vi "Main Engine Stream Process.vi"(8 "error in (no error)":errorcluster, 10 "Refs":T1 {"Port Settings"."FD ISO Mode" items=["ISO", "Non ISO", "ISO Legacy"]; "Port Settings"."Termination" items=["Off", "On"]; "Port Settings"."Mode" items=["CAN 2.0", "CAN FD", "CAN FD+BRS"]}, 11 "Process in":refnum<class "Process.lvclass">=refnum) -> (0 "error out":errorcluster)   [LabVIEW 2021, in "CAN Stream Support Engine.lvlib"]
uses:
  CAN Stream Support Engine.lvlib
  Types/Engine Stream State.ctl
  <vilib>/xnet/xnet.llb/XNET Frame Type CAN.ctl
  <vilib>/xnet/xnet.llb/XNET Frame CAN.ctl
  <resource>/objmgr/xnet.rc
  <vilib>/xnet/xnet.llb/XNET CAN Last Err.ctl
  <vilib>/xnet/xnet.llb/XNET CAN Comm State.ctl
  <vilib>/xnet/xnet.llb/XNET CAN Comm.ctl
  Addon Shared/Types/Stream Type.ctl
  Addon Shared/CAN Stream Support Shared.lvlib
  <vilib>/xnet/xnet.llb/XNET Create Session (Frame Input Stream).vi
  <vilib>/xnet/xnet.llb/XNET Read (State CAN Comm).vi
  <vilib>/xnet/xnet.llb/XNET Read (Frame CAN).vi
  <vilib>/NI/NIVS Inline Async API/_VS Inline Async API/Process/Process.lvclass
  Types/Engine Stream Refs.ctl
  Addon Shared/Types/Type Filter.ctl
  Addon Shared/Types/Direction Filter.ctl
  Addon Shared/Types/Filter Parameters.ctl
  Types/Engine Stream Port Settings.ctl
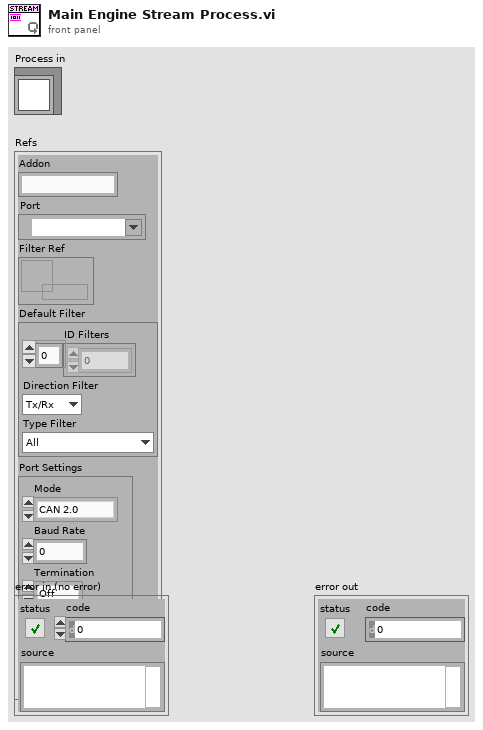
[diagram p1: front panel]
types:
  T1 = typedef "CAN Stream Support Engine.lvlib/Engine Stream Refs.ctl" = cluster{"Addon":string, "Port":refnum<k21>, "Filter Ref":refnum<data-value>, "Default Filter":T2, "Port Settings":T5}
  T2 = typedef "CAN Stream Support Shared.lvlib/Filter Parameters.ctl" = cluster{"ID Filters":u32[], "Direction Filter":T3, "Type Filter":T4}
  T3 = typedef "CAN Stream Support Shared.lvlib/Direction Filter.ctl" = enum16{"Tx/Rx", "Rx", "Tx"}
  T4 = typedef "CAN Stream Support Shared.lvlib/Type Filter.ctl" = enum16{"All", "CAN Data", "CAN Remote", "CAN Bus Error", "CAN 2.0 Data", "CAN FD Data", "CAN FD+BRS Data", "J1939 Data", "Delay", "Log Trigger", "Start Trigger"}
  T5 = typedef "CAN Stream Support Engine.lvlib/Engine Stream Port Settings.ctl" = cluster{"Mode":u32, "Baud Rate":u64, "Termination":u32, "FD ISO Mode":u32, "FD Baud Rate":u64}
  T6 = typedef "CAN Stream Support Engine.lvlib/Engine Stream State.ctl" = enum8{"Check for Connection", "Open XNET Session", "Publish", "Cleanup", "Exit"}
  T7 = typedef "CAN Stream Support Shared.lvlib/Stream Type.ctl" = cluster{"State":T8, "Frames":T11[]}
  T8 = typedef "XNET CAN Comm.ctl" = cluster{"fault code":i32, "fault?":bool, "communication state":T9, "last error":T10, "receive error counter":u8, "transmit error counter":u8, "transceiver error?":bool, "sleep?":bool}
  T9 = typedef "XNET CAN Comm State.ctl" = u8
  T10 = typedef "XNET CAN Last Err.ctl" = u8
  T11 = typedef "XNET Frame CAN.ctl" = cluster{"timestamp":timestamp, "payload":u8[], "identifier":u32, "type":T12, "extended?":bool, "echo?":bool}
  T12 = typedef "XNET Frame Type CAN.ctl" = u8
  T13 = cluster{"ID Filters":u32[], "Direction Filter":T3, "Type Filter":T4}
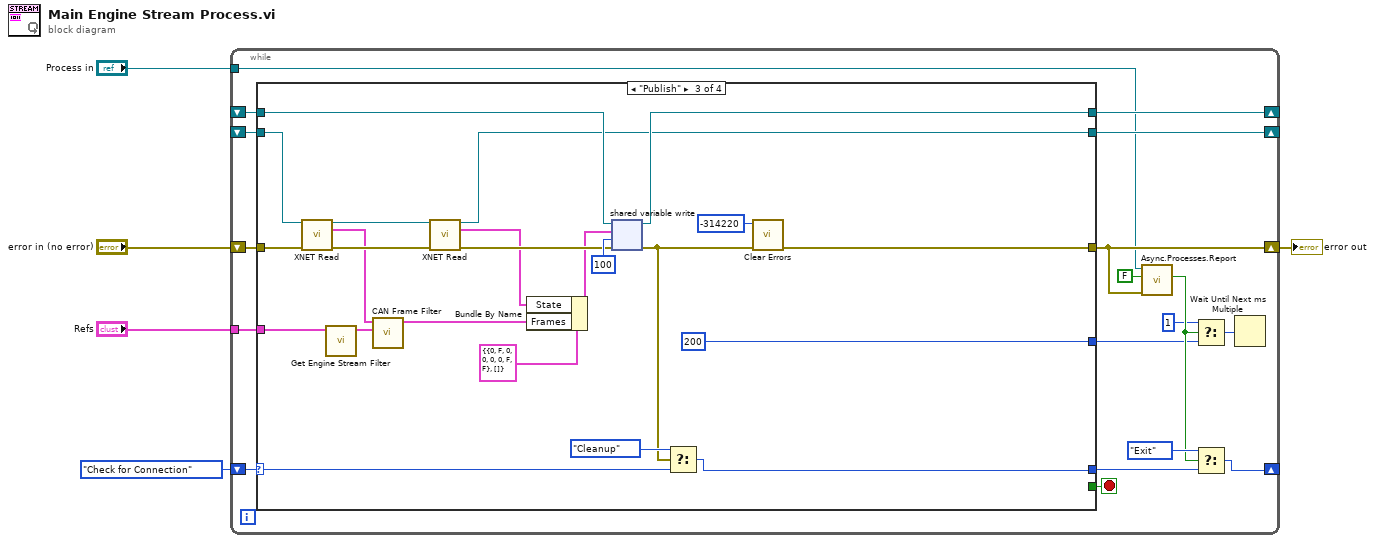
[diagram p0: block diagram]
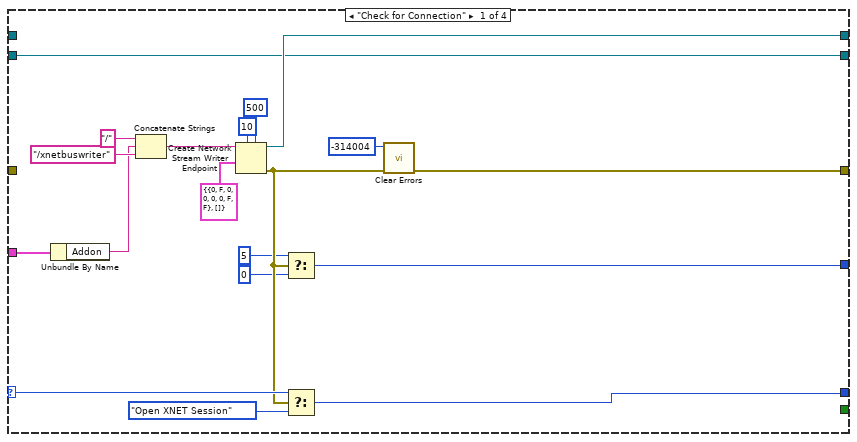
[diagram p2: hidden frame]
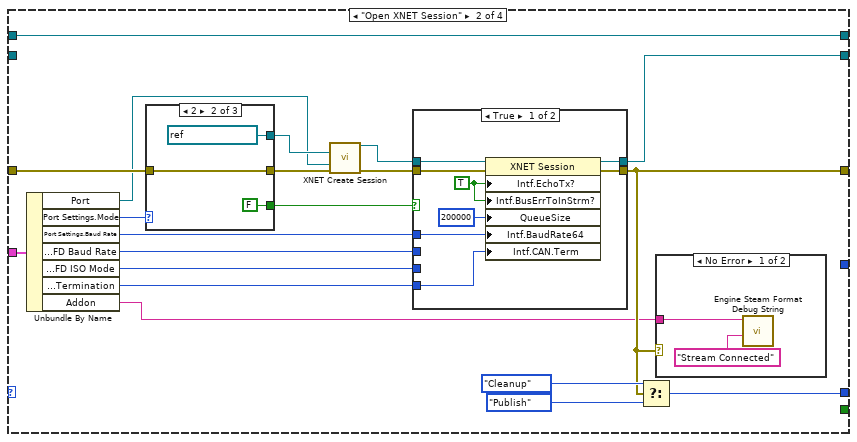
[diagram p3: hidden frame]
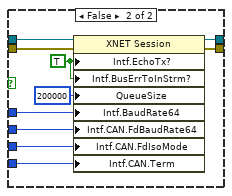
[diagram p4: hidden frame]
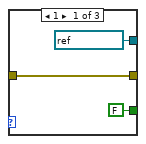
[diagram p5: hidden frame]
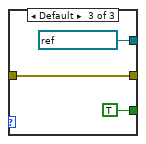
[diagram p6: hidden frame]
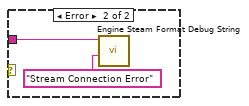
[diagram p7: hidden frame]
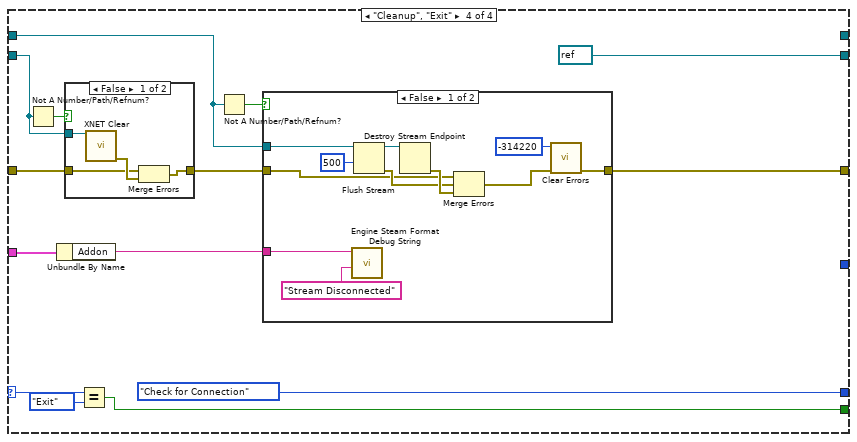
[diagram p8: hidden frame]
diagram:
  n1 = while {
    shift-right: [w11] -> _
    shift-left: Engine_Stream_State."Check for Connection" -> [w23]
    shift-right: [w22] -> _
    shift-left: _ -> [w21]
    shift-right: [w16] -> w3
    shift-left: "error in (no error)" -> [w20]
    shift-right: [w18] -> _
    shift-left: _ -> [w17]
    tunnel: "Process in" -> [w13]
    tunnel: "Refs" -> [w12]
    stop <- w19 stop-if-true
    n2 = case shown="\"Publish\"" w23 {
      selector: w23 -> [w40 _ w113 w129]
      tunnel: [w38 w59 w112 Engine_Stream_State."Check for Connection"] -> w14
      tunnel: [w37 w60 w114 _] -> w22
      tunnel: w21 -> [_ w60 w115 w126]
      tunnel: [w35 w55 w97 w119] -> w16
      tunnel: w20 -> [_ w46 w108 w121]
      tunnel: [_ _ _ w127] -> w19
      tunnel: [w36 w57 w103 refnum<k21> refnum ("session out")] -> w18
      tunnel: w17 -> [w36 _ w110 w123]
      tunnel: [w29 _ u32 200 ("millisecond multiple") _] -> w9
      tunnel: w12 -> [w25 w54 w107 w118]
      frame "Check for Connection" {
        n3 = Unbundle By Name(w25) -> ("Addon"=w24:string)
        n4 = Concatenate Strings("/" ("string"), w24, "/xnetbuswriter" ("reader url")) -> (w26:string)
        n5 = Create Network Stream Writer Endpoint(5:500 ("timeout in ms (-1)"), 7:10 ("writer buffer size"), 9:T7 {"State"={"fault code"=0, "fault?"=FALSE, "communication state"=0, "last error"=0, "receive error counter"=0, "transmit error counter"=0, "transceiver error?"=FALSE, "sleep?"=FALSE}, "Frames"=[]} ("Stream"), 11:w26) -> (0:w32:errorcluster, 3:w37:refnum<k21>)  [unwired: 3 in]
        n6 = Select(t=u32 5 ("millisecond multiple"), s=w32, f=u32 0) -> (s? t:f=w29:u32)
        n7 = Select(t=w40, s=w32, f=Engine_Stream_State."Open XNET Session") -> (s? t:f=w38:T6)
        n8 = call <vilib>:"Clear Errors.vi"("error in (no error)"=w32, "specific error code to clear (0: all)"=-314004) -> ("error out"=w35:errorcluster)  [unwired: 4 in, 1 out]
      }
      frame "Open XNET Session" {
        n9 = Unbundle By Name(w54) -> ("Port"=w43:refnum<k21>, "Port Settings.Mode"=w47:u32, "Port Settings.Baud Rate"=w45:u64, "Port Settings.FD Baud Rate"=w44:u64, "Port Settings.FD ISO Mode"=w48:u32, "Port Settings.Termination"=w52:u32, "Addon"=w53:string)
        n10 = case shown="2" w47 {
          tunnel: [refnum<k21> ":can_fd:" ("cluster (:memory:)") refnum<k21> ":can_fd_brs:" ("cluster (:memory:)") refnum<k21> ":memory:" ("cluster (:memory:)")] -> w51
          tunnel: w46 -> [w81 w84 w87]
          tunnel: [w81 w84 w87] -> w50
          tunnel: [FALSE FALSE TRUE] -> w49
          frame 1 {
          }
          frame 2 {
          }
          frame Default {
          }
        }
        n11 = call-poly <vilib>:"XNET Create Session.vi"("cluster (:memory:)"=w51, "interface"=w43, "error in (no error)"=w50) -> ("session out"=w58:refnum<k21>, "error out"=w56:errorcluster)  [unwired: 11 out]
        n12 = case shown="True" w49 {
          tunnel: w58 -> [w70 w80]
          tunnel: [w69 w79] -> w57
          tunnel: w56 -> [w68 w78]
          tunnel: [w67 w77] -> w55
          tunnel: w52 -> [w64 w74]
          tunnel: w45 -> [w63 w73]
          tunnel: w48 -> [_ w72]
          tunnel: w44 -> [_ w71]
          frame True {
            w65 = TRUE ("Interface:Echo Transmit?")
            n13 = property class="XNET Session"(reference=w70, error in=w68, "Intf.EchoTx?"=w65, "Intf.BusErrToInStrm?"=w65, "QueueSize"=u32 200000 ("Queue Size"), "Intf.BaudRate64"=w63, "Intf.CAN.Term"=w64) -> (reference out=w69:refnum<k21>, error out=w67:errorcluster)
          }
          frame False {
            w75 = TRUE ("Interface:Echo Transmit?")
            n14 = property class="XNET Session"(reference=w80, error in=w78, "Intf.EchoTx?"=w75, "Intf.BusErrToInStrm?"=w75, "QueueSize"=u32 200000 ("Queue Size"), "Intf.BaudRate64"=w73, "Intf.CAN.FdBaudRate64"=w71, "Intf.CAN.FdIsoMode"=w72, "Intf.CAN.Term"=w74) -> (reference out=w79:refnum<k21>, error out=w77:errorcluster)
          }
        }
        n15 = Select(t=Engine_Stream_State."Cleanup", s=w55, f=Engine_Stream_State."Publish") -> (s? t:f=w59:T6)
        n16 = case shown="No Error" w55 {
          tunnel: w53 -> [w90 w92]
          frame No Error {
            n17 = call "Engine Steam Format Debug String.vi"("State"="Stream Connected", "Name"=w90) -> ()  [unwired: 9 in, 1 out]
          }
          frame Error {
            n18 = call "Engine Steam Format Debug String.vi"("State"="Stream Connection Error", "Name"=w92) -> ()  [unwired: 9 in, 1 out]
          }
        }
      }
      frame "Publish" {
        n19 = call-poly <vilib>:"XNET Read.vi"("session in"=w110, "error in (no error)"=w108) -> ("session out"=w104:refnum<k21>, "data"=w96:T11[], "error out"=w106:errorcluster)  [unwired: 11 out]
        n20 = call "Get Engine Stream Filter.vi"("Refs"=w107) -> ("Filter"=w94:T13)  [unwired: 9 in, 1 out]
        n21 = call "CAN Frame Filter.vi"("Filter"=w94, "frames in"=w96) -> ("frames out"=w95:T11[])  [unwired: 9 in]
        n22 = call-poly <vilib>:"XNET Read.vi"("session in"=w104, "error in (no error)"=w106) -> ("session out"=w103:refnum<k21>, "CAN comm"=w102:T8, "error out"=w105:errorcluster)  [unwired: 11 out]
        n23 = Bundle By Name(cluster=T7 {"State"={"fault code"=0, "fault?"=FALSE, "communication state"=0, "last error"=0, "receive error counter"=0, "transmit error counter"=0, "transceiver error?"=FALSE, "sleep?"=FALSE}, "Frames"=[]} ("Stream"), "State"=w102, "Frames"=w95) -> (w101:T7)
        n24 = shared-variable-write(w115, w105, w101, 100 ("timeout ms")) -> (w114:refnum<k21>, w98:errorcluster)  [unwired: 1 out]
        n25 = Select(t=Engine_Stream_State."Cleanup", s=w98, f=w113) -> (s? t:f=w112:T6)
        n26 = call <vilib>:"Clear Errors.vi"("error in (no error)"=w98, "specific error code to clear (0: all)"=-314220) -> ("error out"=w97:errorcluster)  [unwired: 4 in, 1 out]
      }
      frame "Cleanup", "Exit" {
        n27 = Not A Number/Path/Refnum?(number/path/refnum=w123) -> (NaN/Path/Refnum?=w122:bool)
        n28 = Unbundle By Name(w118) -> ("Addon"=w117:string)
        n29 = case shown="False" w122 {
          tunnel: w121 -> [w131 w135]
          tunnel: [w132 w135] -> w120
          tunnel: w123 -> [w134 _]
          frame False {
            n30 = call <vilib>:"XNET Clear.vi"("session in"=w134) -> ("error out"=w133:errorcluster)  [unwired: 14 in]
            n31 = Merge Errors(w131, w133) -> (w132:errorcluster)
          }
          frame True {
          }
        }
        n32 = Equal?(x=w129, y=Engine_Stream_State."Exit") -> (x = y?=w127:bool)
        n33 = Not A Number/Path/Refnum?(number/path/refnum=w126) -> (NaN/Path/Refnum?=w125:bool)
        n34 = case shown="False" w125 {
          tunnel: w120 -> [w139 w147]
          tunnel: [w136 w147] -> w119
          tunnel: w126 -> [w145 _]
          tunnel: w117 -> [w143 _]
          frame False {
            n35 = call "Engine Steam Format Debug String.vi"("State"="Stream Disconnected", "Name"=w143) -> ()  [unwired: 9 in, 1 out]
            n36 = Flush Stream(9:500 ("timeout in ms (-1)"), 11:w145) -> (0:w140:errorcluster, 3:w146:refnum<k21>)  [unwired: 2 in, 1 out]
            n37 = Destroy Stream Endpoint(11:w146) -> (0:w142:errorcluster)  [unwired: 1 in]
            n38 = Merge Errors(w139, w140, w142) -> (w137:errorcluster)
            n39 = call <vilib>:"Clear Errors.vi"("error in (no error)"=w137, "specific error code to clear (0: all)"=-314220) -> ("error out"=w136:errorcluster)  [unwired: 4 in, 1 out]
          }
          frame True {
          }
        }
      }
    }
    n40 = call <vilib>:"Async.Processes.Report.vi"("Error"=w16, "Stop Async on Error?"=FALSE, "Process in"=w13) -> ("Stop"=w10:bool)  [unwired: 7 in, 1 out]
    n41 = Select(t=u32 1, s=w10, f=w9) -> (s? t:f=w8:u32)
    n42 = Select(t=Engine_Stream_State."Exit" ("y"), s=w10, f=w14) -> (s? t:f=w11:T6)
    n43 = Wait Until Next ms Multiple(millisecond multiple=w8) -> ()  [unwired: 1 out]
  }
  "error out" <- w3
